vi "4.6.2.vi"() -> ()   [LabVIEW 2017]
panel:
  in  "停止":bool
  out "结果":dbl
  in  "B":dbl
  in  "A":dbl
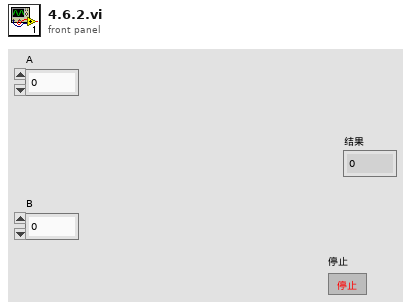
[diagram p1: front panel]
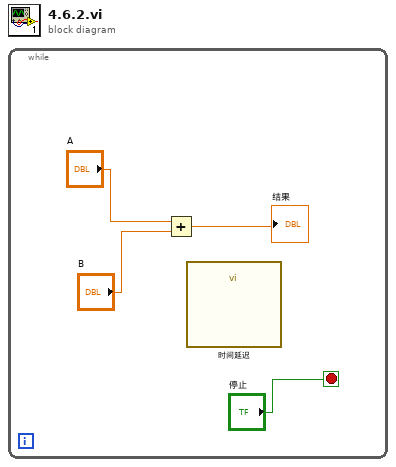
[diagram p0: block diagram]
diagram:
  n1 = while {
    stop <- "停止" stop-if-true
    n2 = Add(x="A", y="B") -> (x+y=→"结果":dbl)
    n3 = call "时间延迟"() -> ()  [unwired: 11 in, 1 out]
  }
